vi "Serial to Float.vi"() -> ()   [LabVIEW 2016]
uses:
  <vilib>/Instr/_visa.llb/VISA Configure Serial Port (Instr).vi
panel:
  in  "byte count":u32
  in  "VISA resource name":refnum<visa-resource-name>
  out "read buffer":string
  out "Array":dbl[][](array[numeric])
  in  "stop 2":bool
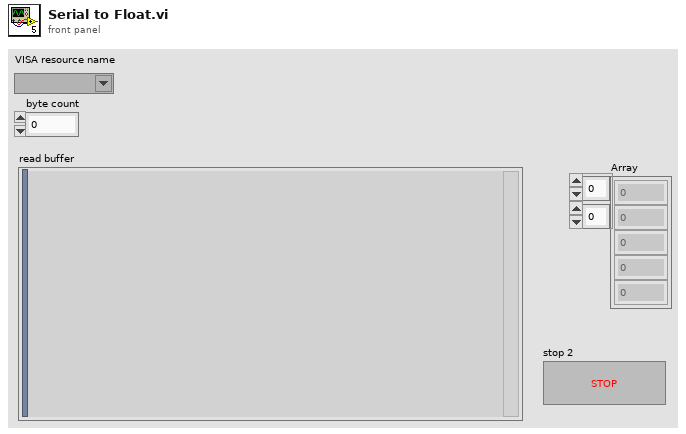
[diagram p1: front panel]
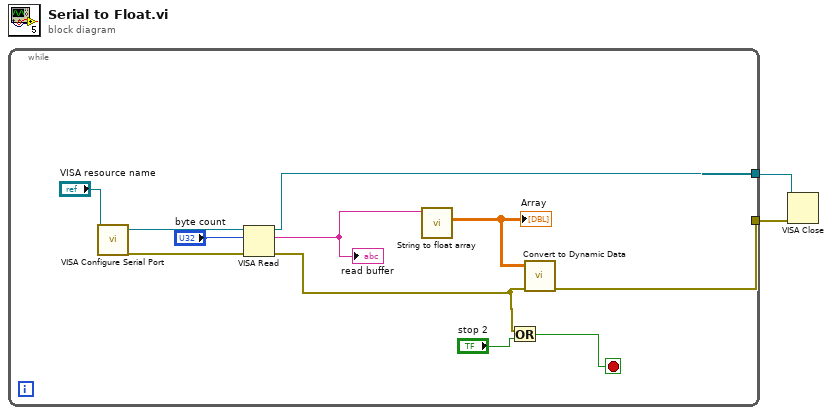
[diagram p0: block diagram]
diagram:
  n1 = while {
    tunnel: [w7] -> w2
    tunnel: [w3] -> w1
    stop <- w5 stop-if-true
    n2 = call-poly "VISA Configure Serial Port"("VISA resource name"="VISA resource name") -> ("VISA resource name out"=w12:refnum<visa-resource-name>, "error out"=w11:errorcluster)  [unwired: 13 in]
    n3 = VISA Read(VISA resource name=w12, byte count="byte count", error in (no error)=w11) -> (VISA resource name out=w7:refnum<visa-resource-name>, read buffer=w8:string, error out=w3:errorcluster)  [unwired: 1 out]
    "read buffer" <- w8
    n4 = call "String to float array.vi"("String"=w8) -> ("Array"=w6:dbl[][])  [unwired: 10 in]
    "Array" <- w6
    n5 = Or(x=w3, y="stop 2") -> (x .or. y?=w5:bool)
    n6 = call "Convert to Dynamic Data"("2D Array"=w6) -> ()  [unwired: 3 in, 1 out]
  }
  n7 = VISA Close(VISA resource name=w2, error in (no error)=w1) -> ()  [unwired: 1 out]
